vi "WhichVIsShouldRegenerate.vi"(10 "CommandTemplatesFolder":path=path "C:/Users/Bendethic/Documents/LabVIEW Data/Projects/xml-auto-routine/CreateCommands/CommandTemplates", 11 "LastModifiedDatesFolder":path=path "C:/Users/Bendethic/Documents/LabVIEW Data/Projects/xml-auto-routine/CreateCommands") -> (2 "iniRefecence":T1, 3 "VINames":string[](array[string]))   [LabVIEW 2017]
uses:
  <vilib>/Utility/config.llb/Config Data RefNum.ctl
  <vilib>/Utility/config.llb/Read Key (String).vi
  <vilib>/Utility/config.llb/NI_LVConfig.lvlib
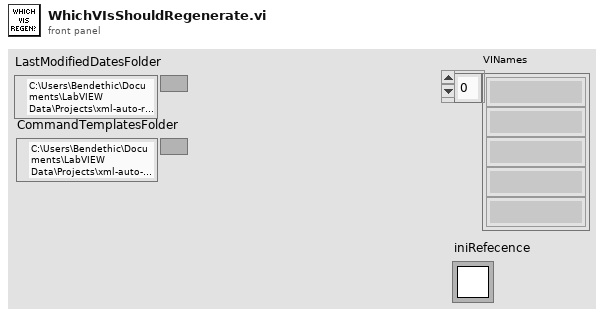
[diagram p1: front panel]
types:
  T1 = typedef "NI_LVConfig.lvlib/Config Data RefNum.ctl" = refnum<k1>
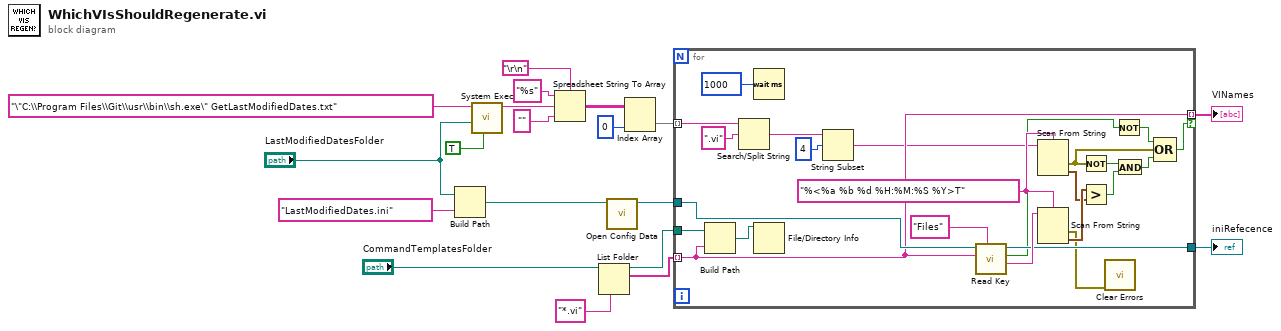
[diagram p0: block diagram]
diagram:
  n1 = Build Path(base path="LastModifiedDatesFolder", name or relative path="LastModifiedDates.ini") -> (appended path=w13:path)
  n2 = call <vilib>:"System Exec.vi"("run minimized? (F)"=TRUE, "working directory"="LastModifiedDatesFolder", "command line"="\"C:\\Program Files\\Git\\usr\\bin\\sh.exe\" GetLastModifiedDates.txt") -> ("standard output"=w6:string)  [unwired: 5 in, 3 out]
  n3 = Spreadsheet String To Array(delimiter (Tab)="\r\n", format string="%s", spreadsheet string=w6, array type (2D Dbl)="" ("format string")) -> (array=w3:string[][])
  n4 = List Folder(path="CommandTemplatesFolder", pattern="*.vi") -> (path out=w10:path, filenames=w11:string[])  [unwired: 2 in, 2 out]
  n5 = call <vilib>:"Open Config Data.vi"("configuration file path"=w13) -> ("refnum"=w9:T1)  [unwired: 8 in, 2 out]
  n6 = Index Array(array=w3, index (col)=0 ("disabled index (col)")) -> (element=w1:string[])  [unwired: 1 in]
  n7 = for {
    tunnel: w11 -> [w37] mode=indexing
    tunnel: w10 -> [w39]
    tunnel: w9 -> [w38]
    tunnel: [w37] -> w8 mode=indexing if=w21
    tunnel: [w36] -> w7
    tunnel: w1 -> [w31] mode=indexing
    w42 = "%<%a %b %d %H:%M:%S %Y>T" ("format string")
    n8 = Build Path(base path=w39, name or relative path=w37) -> (appended path=w40:path)
    n9 = Search/Split String(string=w31, search string/char (-)=".vi") -> (match + rest of string=w33:string)  [unwired: 1 in, 2 out]
    n10 = Wait (ms)(milliseconds to wait=u32 1000) -> ()  [unwired: 1 out]
    n11 = File/Directory Info(path=w40) -> ()  [unwired: 1 in, 7 out]
    n12 = String Subset(string=w33, offset (0)=4) -> (substring=w32:string)  [unwired: 1 in]
    n13 = call-poly <vilib>:"Read Key.vi"("section"="Files", "key"=w37, "refnum"=w38) -> ("value"=w43:string, "found?"=w29:bool, "refnum out"=w36:T1)  [unwired: 5 in, 1 out]
    n14 = Scan From String(format string=w42, input string=w32) -> (error out=w23:errorcluster, output 1=w27:timestamp)  [unwired: 3 in, 2 out]
    n15 = Scan From String(format string=w42, input string=w43) -> (error out=w20:errorcluster, output 1=w28:timestamp)  [unwired: 3 in, 2 out]
    n16 = Not(x=w23) -> (.not. x?=w25:bool)
    n17 = Greater?(x=w28, y=w27) -> (0:w26:bool)
    n18 = call <vilib>:"Clear Errors.vi"("error in (no error)"=w20) -> ()  [unwired: 5 in, 2 out]
    n19 = Not(x=w29) -> (.not. x?=w24:bool)
    n20 = And(x=w25, y=w26) -> (x .and. y?=w22:bool)
    n21 = Compound Arithmetic op=OR(w24, w23, w22) -> (w21:bool)
  }
  "VINames" <- w8
  "iniRefecence" <- w7
